vi "Main.vi"(11 "Module Admin":refnum<class "Delacor_lib_QMH_Module Admin.lvclass">) -> ()   [LabVIEW 2025, in "Logger.lvlib"]
doc: "This template is based off of the Queued Message Handler design pattern and the Queued Message Handler project template that ships with LabVIEW.\n\nThe main difference is that the queue is private to this module and communication between modules is performed via Broadcast and Request events.\n\nRequest events are wrapped in public API methods and are handled in the Event Handling Loop (EHL) of this VI. Any module can register for Broadcast events sent by this module. The EHL generates messages based on user interface actions.\n\nThe Message Handling Loop (MHL) processes messages generated by the EHL, or by other messages. The messages are string values, so new messages can be added easily to the Message Cases case structure in the MHL. Each message cluster can also provide an optional value for Message Data, which is a variant that can be converted to whatever message-specific data is required.\n_____\nBased on DQMH Project Template 4.0.0.47.\n_____\nBased on DQMH Dev Tools: Project Template 7.1.0.1503."
uses:
  Logger.lvlib
  <vilib>/Delacor/Delacor QMH/Libraries/Module Admin_class/Delacor_lib_QMH_Module Admin.lvclass
  Module Data--cluster.ctl
  Stop Argument--cluster.ctl
  <vilib>/Delacor/Delacor QMH/Libraries/Message Queue_class/Delacor_lib_QMH_Message Queue.lvclass/Delacor_lib_QMH_Message Queue.ctl
  <vilib>/Delacor/Delacor QMH/Libraries/Module Admin_class/Delacor_lib_QMH_Module Admin.lvclass/Delacor_lib_QMH_Module Admin.ctl
  Initialize File Argument--cluster.ctl
  Initialize File (Reply Payload)--cluster.ctl
  Log Data Argument--cluster.ctl
  Stop Logging Argument--cluster.ctl
  Settings Editor/Update Application Settings (Reply Payload)--cluster.ctl
  Settings Editor/Settings--cluster.ctl
  Settings Editor/Test Meta Data.ctl
  <vilib>/Utility/miscctls.llb/LVPointTypeDef.ctl
  <vilib>/Delacor/Delacor QMH/Libraries/Message Queue_class/Delacor_lib_QMH_Enqueue Message (Single).vi
  <vilib>/Delacor/Delacor QMH/Libraries/Module Admin_class/Delacor_lib_QMH_Get External Launch.vi
  <vilib>/Delacor/Delacor QMH/Libraries/Message Queue_class/Delacor_lib_QMH_Message Queue.lvclass
  Settings Editor/Settings Editor.lvlib
panel:
  out "Settings":T1
  out "error out":errorcluster
  # "This is a headless module. Show its panel to confirm that the Settings are updated correctly and other debugging tasks. Use the Settings Editor to change the settings for this module."
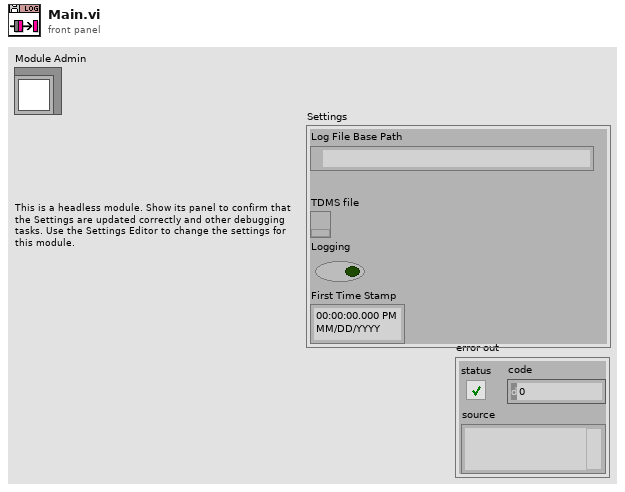
[diagram p1: front panel]
types:
  T1 = typedef "Logger.lvlib/Module Data--cluster.ctl" = cluster{"Log File Base Path":path, "TDMS file":refnum<k34>, "Logging":bool, "First Time Stamp":timestamp}
  T2 = typedef "Settings Editor.lvlib/Broadcast Events--cluster.ctl" = cluster{"Module Did Init":refnum<user-event>, "Status Updated":refnum<user-event>, "Error Reported":refnum<user-event>, "Module Did Stop":refnum<user-event>, "Update Module Execution Status":refnum<user-event>, "Application Settings Updated":refnum<user-event>}
  T3 = typedef "Logger.lvlib/Request Events--cluster.ctl" = cluster{"Stop Module":refnum<user-event>, "Show Panel":refnum<user-event>, "Hide Panel":refnum<user-event>, "Get Module Execution Status":refnum<user-event>, "Show Diagram":refnum<user-event>, "Stop Logging":refnum<user-event>, "Log Data":refnum<user-event>, "Initialize File":refnum<user-event>}
  T4 = enum32{"invalid lock state", "Not Locked", "Locked (No Password)", "Password-protected"}
  T5 = typedef "Logger.lvlib/Stop Argument--cluster.ctl" = cluster{"Origin":string, "Exit via Stop Module Req?":bool, "Wait for Module to stop?":bool}
  T6 = typedef "Logger.lvlib/Initialize File Argument--cluster.ctl" = cluster{"Wait Notifier":refnum<notifier>, "wait for reply":bool}
  T7 = typedef "Logger.lvlib/Log Data Argument--cluster.ctl" = cluster{"Waveform":waveform(dbl)}
  T8 = typedef "Logger.lvlib/Stop Logging Argument--cluster.ctl" = cluster{"Boolean":bool}
  T9 = typedef "Settings Editor.lvlib/Update Application Settings (Reply Payload)--cluster.ctl" = cluster{"Settings":T10, "error":errorcluster}
  T10 = typedef "Settings Editor.lvlib/Settings--cluster.ctl" = cluster{"Log File Base Path":path, "Meta Data":T11, "DAQ Settings":cluster{"physical channel":string, "minimum value":dbl, "maximum value":dbl, "number of samples":i32, "rate":dbl, "custom scale name":string}}
  T11 = typedef "Test Meta Data.ctl" = cluster{"Operator":string, "Job Number":string, "Part Number":string}
  T12 = typedef "LVPointTypeDef.ctl" = cluster{"Horizontal":i16, "Vertical":i16}
  T13 = enum32{"Invalid", "Standard", "Closed", "Hidden", "Minimized", "Maximized"}
  T14 = typedef "Logger.lvlib/Initialize File (Reply Payload)--cluster.ctl" = cluster{"File Path":path, "error":errorcluster}
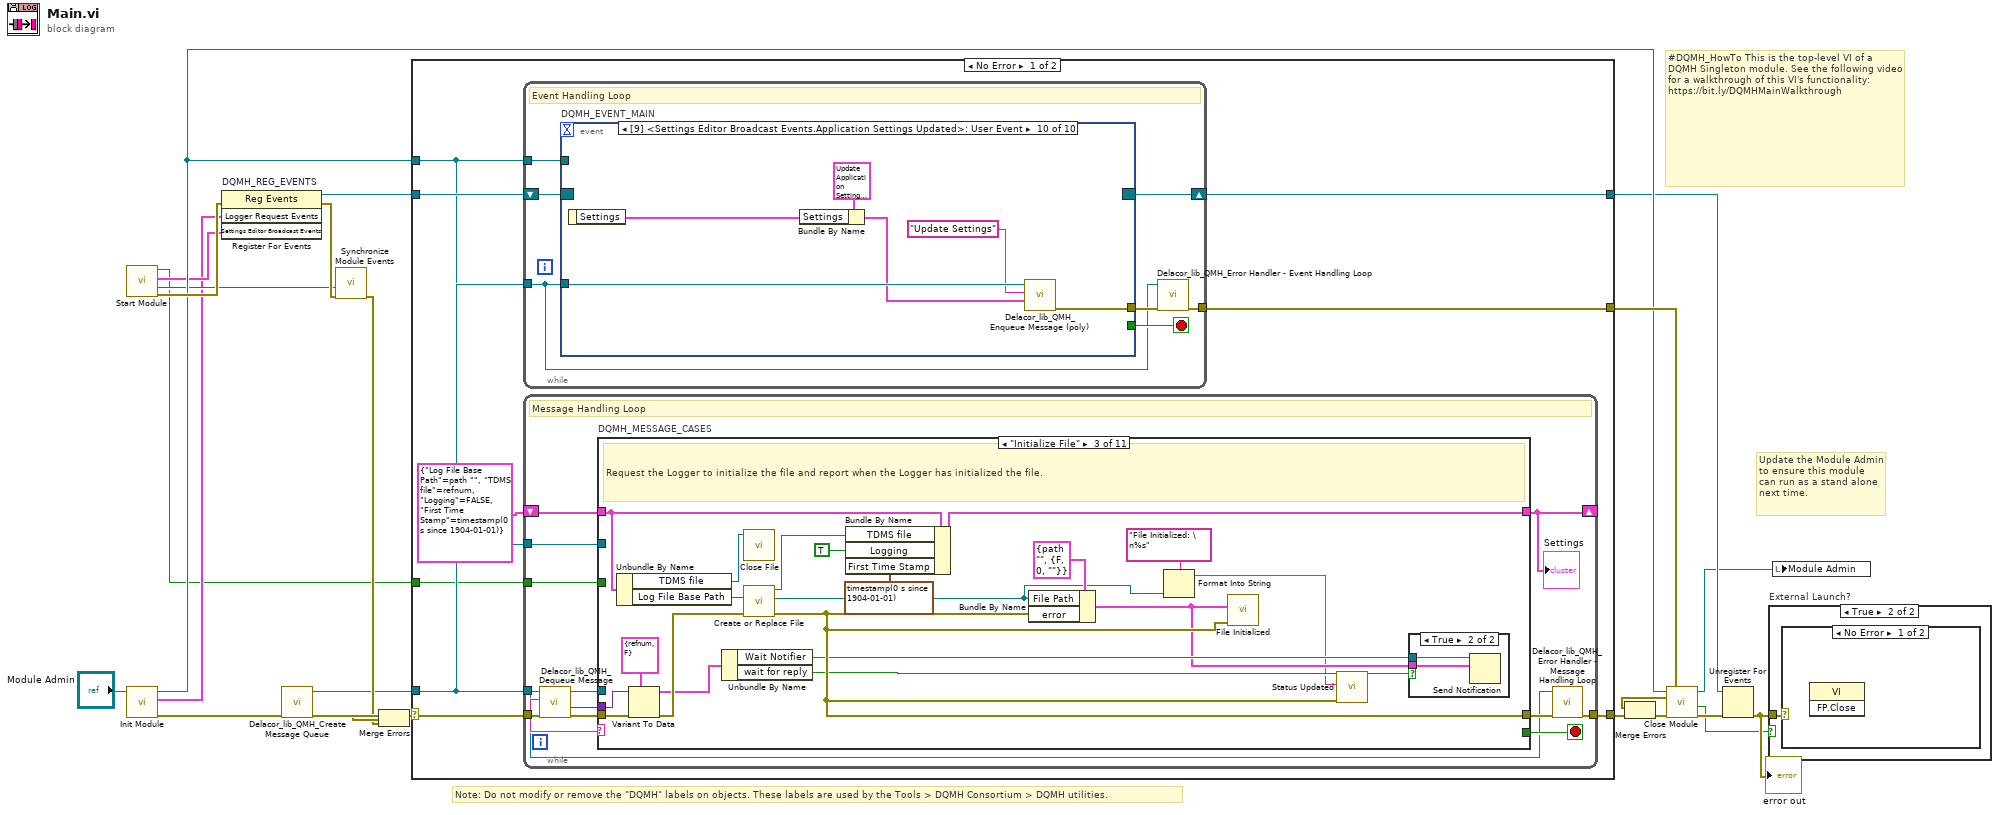
[diagram p0: block diagram]
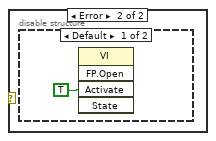
[diagram p3: hidden frame]
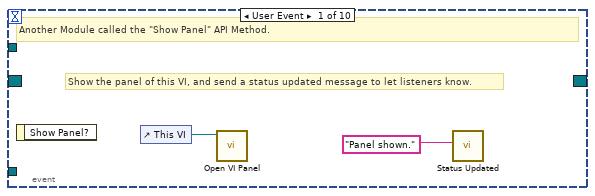
[diagram p5: hidden frame]
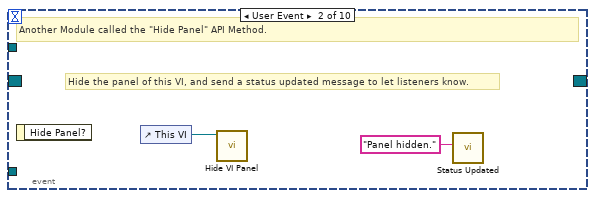
[diagram p6: hidden frame]
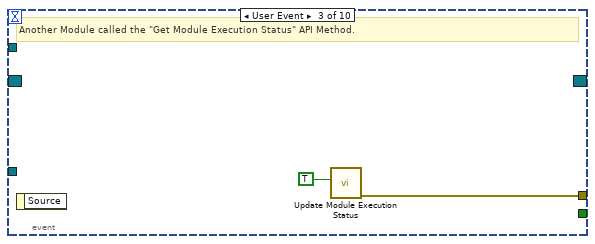
[diagram p7: hidden frame]
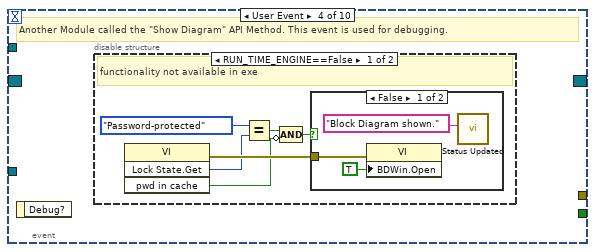
[diagram p8: hidden frame]
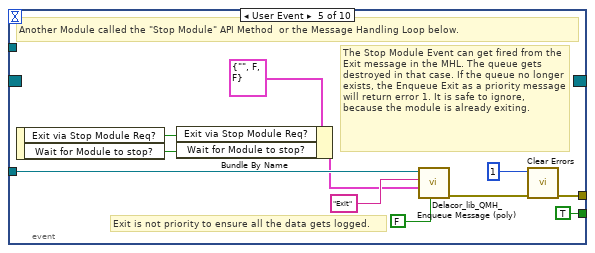
[diagram p11: hidden frame]
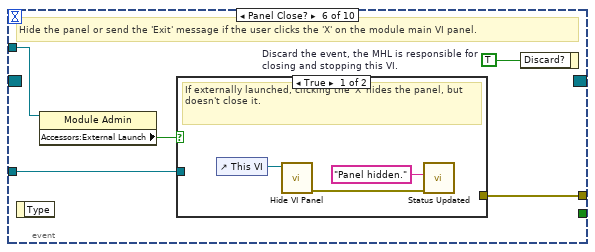
[diagram p12: hidden frame]
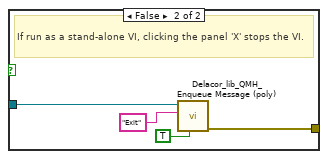
[diagram p13: hidden frame]
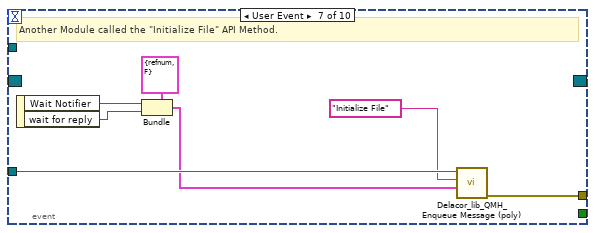
[diagram p14: hidden frame]
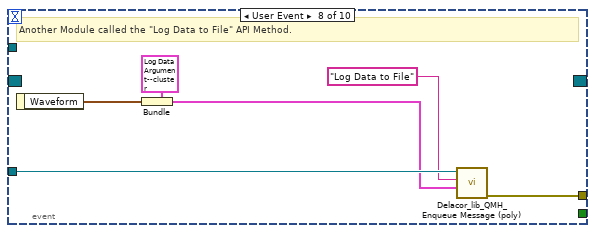
[diagram p15: hidden frame]
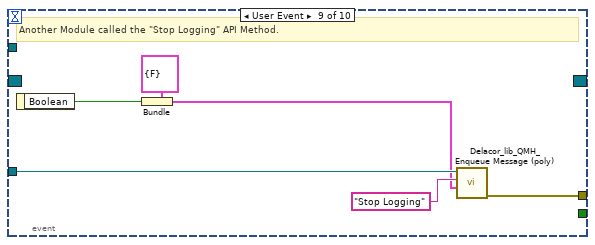
[diagram p16: hidden frame]
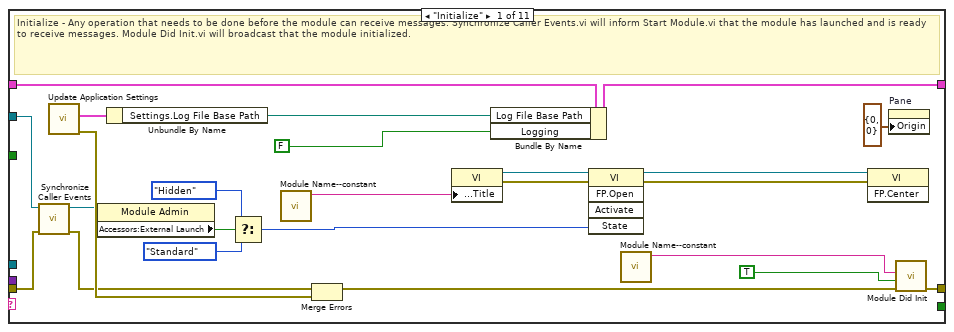
[diagram p17: hidden frame]
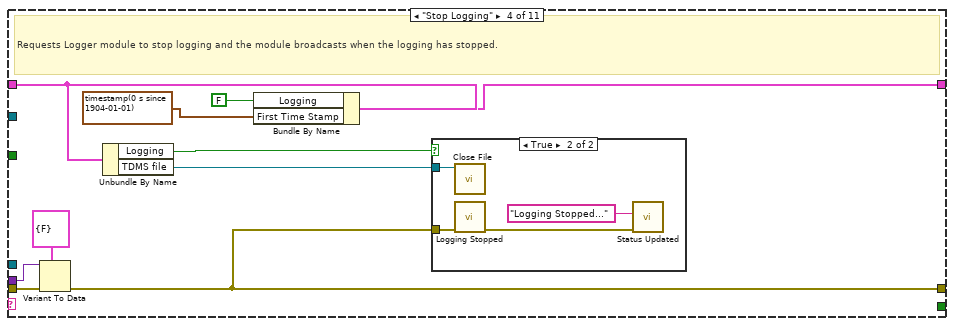
[diagram p20: hidden frame]
diagram:
  # "#DQMH_HowTo This is the top-level VI of a DQMH Singleton module. See the following video for a walkthrough of this VI's functionality: https://bit.ly/DQMHMainWalkthrough"
  # "Note: Do not modify or remove the \"DQMH\" labels on objects. These labels are used by the Tools > DQMH Consortium > DQMH utilities."
  # "Update the Module Admin to ensure this module can run as a stand alone next time."
  n1 = call "Start Module.vi"() -> ("error out"=w14:errorcluster, "Wait for Event Sync?"=w4:bool, "Settings Editor Broadcast Events"=w3:T2, "Module Was Already Running?"=w1:bool)  [unwired: 7 in, 1 out]
  n2 = call "Init Module.vi"("Singleton Module Admin in"="Module Admin") -> ("error out"=w21:errorcluster, "Logger Request Events"=w2:T3, "Singleton Module Admin out"=w11:refnum<class "Delacor_lib_QMH_Module Admin.lvclass">)  [unwired: 8 in]
  n3 = register-events "DQMH_REG_EVENTS"(error in=w14, w2, w3) -> (reference out=w9:refnum<event-registration>, error out=w13:errorcluster)  [unwired: 1 in]
  n4 = call <vilib>:"Delacor_lib_QMH_Create Message Queue.vi"("error in"=w21) -> ("error out"=w16:errorcluster, "Message Queue"=w8:refnum<class "Delacor_lib_QMH_Message Queue.lvclass">)  [unwired: 9 in]
  n5 = call "Synchronize Module Events.vi"("error in"=w13, "Wait for Event Sync?"=w4) -> ("error out"=w12:errorcluster)  [unwired: 9 in]
  n6 = Merge Errors(w16, w12) -> (w15:errorcluster)
  n7 = case shown="No Error" w15 {
    selector: w15 -> [w29 w272]
    tunnel: [w31 w271] -> w22
    tunnel: [w28 w270] -> w10
    tunnel: w9 -> [w26 w270]
    tunnel: w8 -> [w25 w264]
    tunnel: [w30 _] -> w19
    tunnel: w11 -> [w24 w266]
    tunnel: w1 -> [w23 w265]
    frame No Error {
      n8 = while {
        tunnel: w25 -> [w32]
        shift-right: [w35] -> w28
        shift-left: w26 -> [w36]
        tunnel: [w37] -> w30
        tunnel: w24 -> [w33]
        stop <- w34 stop-if-true
        # "Event Handling Loop"
        n9 = event "DQMH_EVENT_MAIN" shown="[9] <Settings Editor Broadcast Events.Application Settings Updated>: User Event" {
          selector: w36 -> [_ _ _ _ _ _ _ _ _ _]
          dyn-events: [_ _ _ _ _ _ _ _ _ _] -> w35
          timeout: _ -> [_ _ _ _ _ _ _ _ _ _]
          tunnel: [_ _ _ _ TRUE ("Discard?") _ _ _ _ _] -> w34
          tunnel: w32 -> [_ _ _ _ w60 w67 w82 w88 w94 w100]
          tunnel: [_ _ w44 _ w63 w69 w83 w89 w95 w101] -> w38
          tunnel: w33 -> [_ _ _ _ _ w66 _ _ _ _]
          event User Event {
            # "Show the panel of this VI, and send a status updated message to let listeners know."
            # "Another Module called the \"Show Panel\" API Method."
            n10 = event-data() -> ()  [unwired: 1 in, 1 out]
            n11 = control-ref of="This VI"() -> (w40:refnum<vi>)
            n12 = call "Open VI Panel.vi"("VI"=w40) -> ()  [unwired: 10 in, 1 out]
            n13 = call "Status Updated.vi"("Status"="Panel shown." ("format string")) -> ()  [unwired: 10 in, 1 out]
          }
          event User Event {
            # "Hide the panel of this VI, and send a status updated message to let listeners know."
            # "Another Module called the \"Hide Panel\" API Method."
            n14 = event-data() -> ()  [unwired: 1 in, 1 out]
            n15 = control-ref of="This VI"() -> (w42:refnum<vi>)
            n16 = call "Hide VI Panel.vi"("VI"=w42) -> ()  [unwired: 10 in, 1 out]
            n17 = call "Status Updated.vi"("Status"="Panel hidden." ("format string")) -> ()  [unwired: 10 in, 1 out]
          }
          event User Event {
            # "Another Module called the \"Get Module Execution Status\" API Method."
            n18 = event-data() -> ()  [unwired: 1 in, 1 out]
            n19 = call "Update Module Execution Status.vi"("Running?"=TRUE) -> ("error out"=w44:errorcluster)  [unwired: 10 in]
          }
          event User Event {
            # "Another Module called the \"Show Diagram\" API Method. This event is used for debugging."
            n20 = event-data() -> ()  [unwired: 1 in, 1 out]
            n21 = disable-structure shown="RUN_TIME_ENGINE==False" {
              frame condition #0 (active) {
                # "functionality not available in exe"
                n22 = invoke on="Invoke Node" class="VI" method="Lock State.Get"() -> (error out=w50:errorcluster, "Get Lock State"=w49:T4, "pwd in cache"=w46:bool)  [unwired: 4 in, 1 out]
                n23 = Equal?(x=T4."Password-protected", y=w49) -> (x = y?=w47:bool)
                n24 = Compound Arithmetic op=AND(w47, invert w46) -> (w45:bool)
                n25 = case shown="False" w45 {
                  tunnel: w50 -> [w53 _]
                  frame False {
                    n26 = property on="Property Node" class="VI"(error in=w53, "BDWin.Open"=TRUE ("Block Diagram Window:Open")) -> ()  [unwired: 1 in, 2 out]
                    n27 = call "Status Updated.vi"("Status"="Block Diagram shown." ("format string")) -> ()  [unwired: 10 in, 1 out]
                  }
                  frame True {
                    # "Password-protected VI, and the password is not in the cache. Do not show the diagram."
                  }
                }
              }
              frame condition #1 {
              }
            }
          }
          event User Event {
            # "Exit is not priority to ensure all the data gets logged."
            # "The Stop Module Event can get fired from the Exit message in the MHL. The queue gets destroyed in that case. If the queue no longer exists, the Enqueue Exit as a priority message will return error 1. It is safe to ignore, because the module is already exiting."
            # "Another Module called the \"Stop Module\" API Method  or the Message Handling Loop below."
            n28 = event-data() -> ("Exit via Stop Module Req?"=w56:bool, "Wait for Module to stop?"=w55:bool)  [unwired: 1 in]
            n29 = Bundle By Name(cluster=T5 {"Origin"="", "Exit via Stop Module Req?"=FALSE, "Wait for Module to stop?"=FALSE} ("Stop Argument"), "Exit via Stop Module Req?"=w56, "Wait for Module to stop?"=w55) -> (w54:T5)
            n30 = call-poly <vilib>:"Delacor_lib_QMH_Enqueue Message (poly).vi"("Priority Message? (F)"=FALSE, "Message Data"=w54, "Message"="Exit", "Message Queue in"=w60) -> ("error out"=w64:errorcluster)  [unwired: 6 in, 1 out]
            n31 = call <vilib>:"Clear Errors.vi"("error in (no error)"=w64, "specific error code to clear (0: all)"=1) -> ("error out"=w63:errorcluster)  [unwired: 4 in, 1 out]
          }
          event Panel Close? {
            w68 = TRUE  # Discard the event, the MHL is responsible for closing and stopping this VI.
            # "Hide the panel or send the 'Exit' message if the user clicks the 'X' on the module main VI panel."
            n32 = event-data() -> ()  [unwired: 1 in, 1 out]
            n33 = property on="Property Node" class="Module Admin"(reference=w66) -> ("Accessors:External Launch"=w65:bool)  [unwired: 1 in, 2 out]
            n34 = case shown="True" w65 {
              tunnel: w67 -> [_ w75]
              tunnel: [_ w76] -> w69
              frame True {
                # "If externally launched, clicking the 'X' hides the panel, but doesn't close it."
                n35 = control-ref of="This VI"() -> (w72:refnum<vi>)
                n36 = call "Hide VI Panel.vi"("VI"=w72) -> ("error out"=w70:errorcluster)  [unwired: 10 in]
                n37 = call "Status Updated.vi"("error in"=w70, "Status"="Panel hidden." ("format string")) -> ()  [unwired: 9 in, 1 out]
              }
              frame False {
                # "If run as a stand-alone VI, clicking the panel 'X' stops the VI."
                n38 = call-poly <vilib>:"Delacor_lib_QMH_Enqueue Message (poly).vi"("Priority Message? (F)"=TRUE, "Message"="Exit", "Message Queue in"=w75) -> ("error out"=w76:errorcluster)  [unwired: 7 in, 1 out]
              }
            }
            n39 = event-data ("Event Filter Node")("Discard?"=w68) -> ()  [unwired: 1 in, 1 out]
          }
          event User Event {
            # "Another Module called the \"Initialize File\" API Method."
            n40 = event-data() -> ("Wait Notifier"=w78:refnum<notifier>, "wait for reply"=w77:bool)  [unwired: 1 in]
            n41 = Bundle(cluster=T6 {"Wait Notifier"=refnum, "wait for reply"=FALSE} ("Initialize File Argument"), "Wait Notifier"=w78, "wait for reply"=w77) -> (w79:T6)
            n42 = call-poly <vilib>:"Delacor_lib_QMH_Enqueue Message (poly).vi"("Message Data"=w79, "Message"="Initialize File", "Message Queue in"=w82) -> ("error out"=w83:errorcluster)  [unwired: 7 in, 1 out]
          }
          event User Event {
            # "Another Module called the \"Log Data to File\" API Method."
            n43 = event-data() -> ("Waveform"=w84:waveform(dbl))  [unwired: 1 in]
            n44 = Bundle(cluster=T7 {"Waveform"={"t0"=timestamp(0 s since 1904-01-01), "dt"=1.0, "Y"=[]}} ("Log Data to File Argument"), "Waveform"=w84) -> (w85:T7)
            n45 = call-poly <vilib>:"Delacor_lib_QMH_Enqueue Message (poly).vi"("Message Data"=w85, "Message"="Log Data to File", "Message Queue in"=w88) -> ("error out"=w89:errorcluster)  [unwired: 7 in, 1 out]
          }
          event User Event {
            # "Another Module called the \"Stop Logging\" API Method."
            n46 = event-data() -> ("Boolean"=w90:bool)  [unwired: 1 in]
            n47 = Bundle(cluster=T8 {"Boolean"=FALSE} ("Stop Logging Argument"), "Boolean"=w90) -> (w91:T8)
            n48 = call-poly <vilib>:"Delacor_lib_QMH_Enqueue Message (poly).vi"("Message Data"=w91, "Message"="Stop Logging", "Message Queue in"=w94) -> ("error out"=w95:errorcluster)  [unwired: 7 in, 1 out]
          }
          event User Event {
            n49 = event-data() -> ("Settings"=w97:T10)  [unwired: 1 in]
            n50 = Bundle By Name(cluster=T9 {"Settings"={"Log File Base Path"=path "", "Meta Data"={"Operator"="", "Job Number"="", "Part Number"=""}, "DAQ Settings"={"physical channel"="cDAQ9181-1913300Mod1/ai0", "minimum value"=0.0, "maximum value"=94400.0, "number of samples"=10, "rate"=125.0, "custom scale name"="Pressure"}}, "error"={"status"=FALSE, "code"=0, "source"=""}} ("Settings Updated Argument"), "Settings"=w97) -> (w96:T9)
            n51 = call-poly <vilib>:"Delacor_lib_QMH_Enqueue Message (poly).vi"("Message Data"=w96, "Message"="Update Settings", "Message Queue in"=w100) -> ("error out"=w101:errorcluster)  [unwired: 7 in, 1 out]
          }
        }
        n52 = call-dynamic "Delacor_lib_QMH_Error Handler - Event Handling Loop.vi"("error in"=w38, "Message Queue in"=w32) -> ("dup error in"=w37:errorcluster)  [unwired: 8 in, 1 out]
      }
      n53 = while {
        tunnel: w25 -> [w105]
        shift-right: [w109] -> _
        shift-left: T1 {"Log File Base Path"=path "", "TDMS file"=refnum, "Logging"=FALSE, "First Time Stamp"=timestamp(0 s since 1904-01-01)} ("Data Cluster") -> [w110]
        tunnel: w29 -> [w113]
        tunnel: [w111] -> w31
        tunnel: w24 -> [w103]
        tunnel: w23 -> [w102]
        stop <- w108 stop-if-true
        # "Message Handling Loop"
        n54 = call-dynamic "Delacor_lib_QMH_Dequeue Message.vi"("error in"=w113, "Message Queue in"=w105) -> ("error out"=w112:errorcluster, "Message Data"=w106:variant, "Message"=w107:string, "Message Queue out"=w104:refnum<class "Delacor_lib_QMH_Message Queue.lvclass">)  [unwired: 6 in]
        n55 = case "DQMH_MESSAGE_CASES" shown="\"Initialize File\"" w107 {
          selector: w107 -> [_ _ _ _ _ _ _ _ _ _ w259]
          tunnel: w104 -> [_ _ _ _ _ _ _ _ w221 w245 _]
          tunnel: w112 -> [w136 w140 w159 w172 w185 w196 w215 w217 w228 w251 w262]
          tunnel: [w115 w140 w160 w171 w184 w194 w214 w217 w224 w246 w263] -> w114
          tunnel: w110 -> [w126 w139 w148 w168 w183 w187 w213 w216 w223 w237 w260]
          tunnel: [w120 w139 w147 w165 w181 w186 w213 w216 w223 w237 w260] -> w109
          tunnel: [_ _ _ _ _ _ _ _ _ w244 _] -> w108
          tunnel: w106 -> [_ _ w157 w170 w182 w193 _ _ w222 w243 _]
          tunnel: w103 -> [w127 _ _ _ _ _ _ _ w220 w238 _]
          tunnel: w102 -> [_ _ _ _ _ _ _ _ _ w235 _]
          frame "Initialize" {
            # "Initialize - Any operation that needs to be done before the module can receive messages. Synchronize Caller Events.vi will inform Start Module.vi that the module has launched and is ready to receive messages. Module Did Init.vi will broadcast that the module initialized."
            n56 = call "Synchronize Caller Events.vi"("error in"=w136, "Singleton Module Admin in"=w127) -> ("error out"=w117:errorcluster, "Singleton Module Admin out"=w123:refnum<class "Delacor_lib_QMH_Module Admin.lvclass">)  [unwired: 8 in]
            n57 = call "Update Application Settings.vi"() -> ("error out"=w135:errorcluster, "Reply Payload"=w121:T9)  [unwired: 9 in, 1 out]
            n58 = property on="Property Node" class="Module Admin"(reference=w123) -> ("Accessors:External Launch"=w131:bool)  [unwired: 1 in, 2 out]
            n59 = Unbundle By Name(w121) -> ("Settings.Log File Base Path"=w119:path)
            n60 = Select(t=T13."Hidden" ("State"), s=w131, f=T13."Standard" ("State")) -> (s? t:f=w128:T13)
            n61 = call "Module Name--constant.vi"() -> ("Module Name"=w134:string)  [unwired: 11 in]
            n62 = Merge Errors(w117, w135) -> (w116:errorcluster)
            n63 = property on="Property Node" class="VI"("Front Panel.Title"=w134) -> (reference out=w133:refnum<vi>, error out=w138:errorcluster)  [unwired: 2 in]
            n64 = Bundle By Name(cluster=w126, "Log File Base Path"=w119, "Logging"=FALSE) -> (w120:T1)
            n65 = invoke on="Invoke Node" class="VI" method="FP.Open"(reference=w133, error in=w138, "State"=w128) -> (reference out=w132:refnum<vi>, error out=w137:errorcluster)  [unwired: 2 in, 3 out]
            n66 = call "Module Name--constant.vi"() -> ("Module Name"=w124:string)  [unwired: 11 in]
            n67 = invoke on="Invoke Node" class="VI" method="FP.Center"(reference=w132, error in=w137) -> ()  [unwired: 1 in, 3 out]
            n68 = property on="Pane" class="Pane"("Origin"=T12 {"Horizontal"=0, "Vertical"=0}) -> ()  [unwired: 2 in, 2 out]
            n69 = call "Module Did Init.vi"("error in"=w116, "Initialized?"=TRUE, "Origin"=w124) -> ("error out"=w115:errorcluster)  [unwired: 8 in]
          }
          frame "---Module Specific---" {
            # "Separator -- The following cases handle messages specific to this Module."
          }
          frame "Initialize File" {
            # "Request the Logger to initialize the file and report when the Logger has initialized the file."
            n70 = Unbundle By Name(w148) -> ("TDMS file"=w145:refnum<k34>, "Log File Base Path"=w150:path)
            n71 = Variant To Data(error in=w159, type=T6 {"Wait Notifier"=refnum, "wait for reply"=FALSE} ("Initialize File Argument"), Variant=w157) -> (data=w155:T6, error out=w158:errorcluster)
            n72 = Unbundle By Name(w155) -> ("Wait Notifier"=w154:refnum<notifier>, "wait for reply"=w153:bool)
            n73 = call "Close File.vi"("Refnum out"=w145) -> ()  [unwired: 10 in, 1 out]
            n74 = call "Create or Replace File.vi"("error in"=w158, "Log File Base Path"=w150) -> ("error out"=w160:errorcluster, "File Path"=w142:path, "Refnum out"=w149:refnum<k34>)  [unwired: 7 in]
            n75 = Bundle By Name(cluster=w148, "TDMS file"=w149, "Logging"=TRUE, "First Time Stamp"=timestamp(0 s since 1904-01-01)) -> (w147:T1)
            n76 = Bundle By Name(cluster=T14 {"File Path"=path "", "error"={"status"=FALSE, "code"=0, "source"=""}} ("Initialize File (Reply Payload)"), "File Path"=w142, "error"=w160) -> (w151:T14)
            n77 = Format Into String(format string="File Initialized: \n%s", w142) -> (resulting string=w141:string)  [unwired: 2 in, 1 out]
            n78 = call "File Initialized.vi"("error in"=w160, "Reply Payload"=w151) -> ()  [unwired: 9 in, 1 out]
            n79 = call "Status Updated.vi"("error in"=w160, "Status"=w141) -> ()  [unwired: 9 in, 1 out]
            n80 = case shown="True" w153 {
              tunnel: w154 -> [_ w162]
              tunnel: w151 -> [_ w161]
              frame False {
              }
              frame True {
                n81 = Send Notification(notification=w161, notifier=w162) -> ()  [unwired: 1 in, 2 out]
              }
            }
          }
          frame "Stop Logging" {
            # "Requests Logger module to stop logging and the module broadcasts when the logging has stopped."
            n82 = Variant To Data(error in=w172, type=T8 {"Boolean"=FALSE} ("Stop Logging Argument"), Variant=w170) -> (error out=w171:errorcluster)  [unwired: 1 out]
            n83 = Unbundle By Name(w168) -> ("Logging"=w167:bool, "TDMS file"=w166:refnum<k34>)
            n84 = Bundle By Name(cluster=w168, "Logging"=FALSE, "First Time Stamp"=timestamp(0 s since 1904-01-01)) -> (w165:T1)
            n85 = case shown="True" w167 {
              tunnel: w171 -> [_ w176]
              tunnel: w166 -> [_ w173]
              frame False {
                # "We were not logging, so this is a no-op."
              }
              frame True {
                n86 = call "Close File.vi"("Refnum out"=w173) -> ()  [unwired: 10 in, 1 out]
                n87 = call "Logging Stopped.vi"("error in"=w176) -> ("error out"=w175:errorcluster)  [unwired: 10 in]
                n88 = call "Status Updated.vi"("error in"=w175, "Status"="Logging Stopped...") -> ()  [unwired: 9 in, 1 out]
              }
            }
          }
          frame "Update Settings" {
            n89 = Variant To Data(error in=w185, type=T9 {"Settings"={"Log File Base Path"=path "", "Meta Data"={"Operator"="", "Job Number"="", "Part Number"=""}, "DAQ Settings"={"physical channel"="cDAQ9181-1913300Mod1/ai0", "minimum value"=0.0, "maximum value"=94400.0, "number of samples"=10, "rate"=125.0, "custom scale name"="Pressure"}}, "error"={"status"=FALSE, "code"=0, "source"=""}} ("Settings Updated Argument"), Variant=w182) -> (data=w180:T9, error out=w184:errorcluster)
            n90 = Unbundle By Name(w180) -> ("Settings.Log File Base Path"=w179:path)
            n91 = Bundle By Name(cluster=w183, "Log File Base Path"=w179) -> (w181:T1)
            n92 = call "Status Updated.vi"("error in"=w184, "Status"="Settings Updated") -> ()  [unwired: 9 in, 1 out]
          }
          frame "Log Data to File" {
            # "Requests Logger module to log data to file"
            n93 = Variant To Data(error in=w196, type=T7 {"Waveform"={"t0"=timestamp(0 s since 1904-01-01), "dt"=1.0, "Y"=[]}} ("Log Data to File Argument"), Variant=w193) -> (data=w191:T7, error out=w195:errorcluster)
            n94 = Unbundle By Name(w187) -> ("Logging"=w188:bool, "TDMS file"=w189:refnum<k34>)
            n95 = Unbundle By Name(w191) -> ("Waveform"=w190:waveform(dbl))
            n96 = case shown="True" w188 {
              tunnel: w195 -> [w198 w207]
              tunnel: [w198 w206] -> w194
              tunnel: w190 -> [_ w199]
              tunnel: w189 -> [_ w205]
              tunnel: w187 -> [w197 w204]
              tunnel: [w197 w200] -> w186
              frame False {
                # "We are not currently logging, so this action is a no-op."
              }
              frame True {
                n97 = Unbundle By Name(w204) -> ("First Time Stamp"=w203:timestamp)
                n98 = Equal?(x=w203, y=timestamp(0 s since 1904-01-01) ("First Time Stamp")) -> (x = y?=w201:bool)
                n99 = case shown="True" w201 {
                  tunnel: w204 -> [w208 w212]
                  tunnel: w199 -> [_ w209]
                  tunnel: [w208 w210] -> w200
                  frame False {
                  }
                  frame True {
                    n100 = Unbundle By Name(w209) -> ("t0"=w211:timestamp)
                    n101 = Bundle By Name(cluster=w212, "First Time Stamp"=w211) -> (w210:T1)
                  }
                }
                n102 = call "Log Data to File.vi"("Data Cluster"=w200, "error in"=w207, "Waveform"=w199, "TDMS File Reference"=w205) -> ("error out"=w206:errorcluster)  [unwired: 7 in]
              }
            }
          }
          frame "---Copy This Frame---" {
            # "Duplicate this frame when creating new messages.  Change this comment in the duplicated frame to describe this message."
            n103 = Merge Errors(w215) -> (w214:errorcluster)
          }
          frame "---Exit and Error Handling---" {
            # "Separator - The following cases handle errors and exit messages."
          }
          frame "Error" {
            # "Error - Check the error message data and respond accordingly. This message is sent by the \"Error Handler\" VIs at the end of each loop in this application."
            n104 = property on="Property Node" class="Module Admin"(reference=w220) -> ("Accessors:External Launch"=w219:bool)  [unwired: 1 in, 2 out]
            n105 = Variant To Data(error in=w228, type=errorcluster {"status"=FALSE, "code"=0, "source"=""} ("error constant"), Variant=w222) -> (data=w218:errorcluster, error out=w226:errorcluster)
            n106 = local write "error out"(w218) -> ()
            n107 = call "Error Reported.vi"("Error"=w218) -> ()  [unwired: 10 in, 1 out]
            n108 = case shown="False" w219 {
              tunnel: [w233 _] -> w225
              tunnel: w221 -> [w231 _]
              tunnel: w218 -> [w232 _]
              frame False {
                n109 = disable-structure shown="Default" {
                  disable-tunnel: w232 -> [w234 _]
                  frame condition #0 (active) {
                    # "If the module is running standalone, then pop up an error dialog and call the \"Exit\" message."
                    n110 = call <vilib>:"Simple Error Handler.vi"("error in (no error)"=w234) -> ()  [unwired: 4 in, 5 out]
                  }
                  frame condition #1 {
                    # "To prevent the Simple Error Handler VI from being loaded (e.g. when deploying to a Real-Time target), add the Conditional Disable Symbol \"DQMH_Disable_SEH\" to your project and set it to TRUE."
                  }
                }
                n111 = call-poly <vilib>:"Delacor_lib_QMH_Enqueue Message (poly).vi"("Priority Message? (F)"=TRUE, "Message"="Exit", "Message Queue in"=w231) -> ("error out"=w233:errorcluster)  [unwired: 7 in, 1 out]
              }
              frame True {
                # "If the module was launched externally, calling the Error Reported broadcast VI is the only action performed by the \"Error\" message. The module's caller can then process the error appropriately."
              }
            }
            n112 = Merge Errors(w226, w225) -> (w224:errorcluster)
          }
          frame "Exit" {
            w244 = TRUE  # Stop the VI
            # "Release the message queue reference"
            # "Exit - Exit the application."
            n113 = Variant To Data(error in=w251, type=T5 {"Origin"="", "Exit via Stop Module Req?"=FALSE, "Wait for Module to stop?"=FALSE} ("Stop Argument"), Variant=w243) -> (data=w240:T5, error out=w248:errorcluster)
            n114 = call <vilib>:"Clear Errors.vi"("error in (no error)"=w248, "specific error code to clear (0: all)"=91 ("91: not all Exit messages will have an argument")) -> ("error out"=w250:errorcluster)  [unwired: 4 in, 1 out]
            n115 = Unbundle By Name(w237) -> ("TDMS file"=w236:refnum<k34>)
            n116 = control-ref of="This VI"() -> (w239:refnum<vi>)
            n117 = call-dynamic "Delacor_lib_QMH_Release Message Queue.vi"("error in"=w250, "Message Queue"=w245) -> ("error out"=w249:errorcluster)  [unwired: 9 in]
            n118 = call "Handle Exit.vi"("Stop Argument"=w240, "Admin in"=w238, "VI reference"=w239) -> ("error out"=w247:errorcluster)  [unwired: 7 in, 1 out]
            n119 = call "Close File.vi"("Refnum out"=w236) -> ()  [unwired: 10 in, 1 out]
            n120 = Merge Errors(w249, w247) -> (w246:errorcluster)
            n121 = case "Settings Editor was\nalready running?" shown="False" w235 {
              frame False {
                n122 = call "Module Name--constant.vi"() -> ("Module Name"=w253:string)  [unwired: 11 in]
                n123 = call "Stop Module.vi"("Wait for Module to Stop? (F)"=TRUE, "Origin"=w253) -> ()  [unwired: 9 in, 1 out]
              }
              frame True {
                # "Another Module is\nin charge of stopping Settings Editor"
              }
            }
            n124 = call "Error Reported.vi"("Error"=w246) -> ()  [unwired: 10 in, 1 out]
          }
          frame Default {
            # "'Default' case only runs if there is a message that isn't defined in any of the other cases.  Output a programming error."
            n125 = call "Module Name--constant.vi"() -> ("Module Name"=w258:string)  [unwired: 11 in]
            n126 = Format Into String(format string="The invalid message string \"%s\" was received in the Message Handling Loop for module \"%s\".", w259, w258) -> (resulting string=w256:string)  [unwired: 2 in, 1 out]
            n127 = call <vilib>:"Error Cluster From Error Code.vi"("show call chain? (False)"=TRUE, "error message (\"\")"=w256, "error code (0)"=1) -> ("error out"=w261:errorcluster)  [unwired: 6 in]
            n128 = Merge Errors(w262, w261) -> (w263:errorcluster)
          }
        }
        "Settings" <- w109
        n129 = call-dynamic "Delacor_lib_QMH_Error Handler - Message Handling Loop.vi"("error in"=w114, "Message Queue in"=w104) -> ("dup error in"=w111:errorcluster)  [unwired: 8 in, 1 out]
      }
    }
    frame Error {
      # "Synchronize Caller Events.vi will inform Start Module.vi that the module has launched and will let the code calling Start Module.vi register for broadcasts and would permit the caller receive the broadcast that an error occurred at launch time."
      n130 = call "Synchronize Caller Events.vi"("Singleton Module Admin in"=w266) -> ("error out"=w273:errorcluster)  [unwired: 9 in, 1 out]
      n131 = call-dynamic "Delacor_lib_QMH_Release Message Queue.vi"("error in"=w272, "Message Queue"=w264) -> ("error out"=w271:errorcluster)  [unwired: 9 in]
      n132 = call "Module Name--constant.vi"() -> ("Module Name"=w269:string)  [unwired: 11 in]
      n133 = case "Settings Editor was\nalready running?" shown="False" w265 {
        frame False {
          n134 = call "Module Name--constant.vi"() -> ("Module Name"=w276:string)  [unwired: 11 in]
          n135 = call "Stop Module.vi"("Wait for Module to Stop? (F)"=TRUE, "Origin"=w276) -> ()  [unwired: 9 in, 1 out]
        }
        frame True {
          # "Another Module is\nin charge of stopping Settings Editor"
        }
      }
      n136 = Format Into String(format string="An error occurred during initialization. %s is no longer running.", w269) -> (resulting string=w267:string)  [unwired: 2 in, 1 out]
      n137 = Merge Errors(w272, w273) -> (w274:errorcluster)
      n138 = call "Error Reported.vi"("Additional Information"=w267, "Error"=w274) -> ()  [unwired: 9 in, 1 out]
    }
  }
  n139 = Merge Errors(w19, w22) -> (w18:errorcluster)
  n140 = call "Close Module.vi"("error in"=w18, "Module Admin in"=w11) -> ("error out"=w20:errorcluster, "External Launch"=w5:bool, "Module Admin out"=w6:refnum<class "Delacor_lib_QMH_Module Admin.lvclass">)  [unwired: 7 in]
  n141 = Unregister For Events(event registration refnum=w10, error in=w20) -> (error out=w17:errorcluster)
  "error out" <- w17
  n142 = case "External Launch?" shown="True" w5 {
    tunnel: w17 -> [_ w277]
    frame False {
    }
    frame True {
      n143 = case shown="No Error" w277 {
        frame No Error {
          n144 = invoke on="Invoke Node" class="VI" method="FP.Close"() -> ()  [unwired: 3 in, 3 out]
        }
        frame Error {
          n145 = disable-structure shown="Default" {
            frame condition #0 (active) {
              n146 = invoke class="VI" method="FP.Open"("Activate"=TRUE ("Activate?")) -> ()  [unwired: 4 in, 5 out]
            }
            frame condition #1 {
              # "Don't show panel on error if running inside a built EXE."
            }
          }
        }
      }
    }
  }
  n147 = local write "Module Admin"(w6) -> ()
